vi "CANOpen Edit PDO.vi"(8 "error in (no error)":errorcluster, 11 "Node Ptr":u64 format="%.0x") -> ()   [LabVIEW 2021, in "CANOpen Addon System Explorer.lvlib"]
uses:
  CANOpen Addon System Explorer.lvlib
  SubVIs/CANOpen_PDO Type.ctl
  Shared/CANOpen Addon GUID Lookup Global.vi
  <vilib>/NI VeriStand/Custom Device API/Get Item Property (Variant).vi
  <vilib>/NI VeriStand/Custom Device API/Custom Device API.lvlib
  Shared/CANOpen Addon Shared.lvlib
  <vilib>/NI VeriStand/Custom Device Tools/Custom Device Utility Library/Custom Device Utility Library.lvlib
panel:
  out "error out":errorcluster
  in  "Tag":string
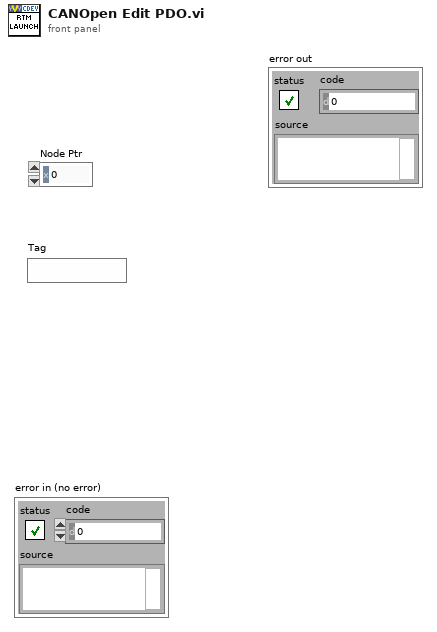
[diagram p1: front panel]
types:
  T1 = typedef "Custom Device API.lvlib/Custom Device Item Info.ctl" = cluster{"Name":string, "Is Channel":bool, "GUID":string, "Is Waveform":bool}
  T2 = typedef "Custom Device API.lvlib/Custom Device Item Ref.ctl" = u64
  T3 = typedef "CANOpen Addon System Explorer.lvlib/CANOpen_PDO Type.ctl" = enum16{"RPDO", "TPDO"}
  T4 = typedef "CANOpen Addon Shared.lvlib/CANOpen_PDO Parameter Settings.ctl" = cluster{"Parameter Name":string, "Scale Factor":dbl, "Scale Offset":dbl, "Byte Offset":u8, "Bit Offset":u8, "Data Type":T5, "Byte Order":T6}
  T5 = typedef "CANOpen Addon Shared.lvlib/CANOpen_PDO Data Type.ctl" = enum16{"U8", "U16", "U32", "I8", "I16", "I32", "Single", "Double", "Boolean"}
  T6 = typedef "CANOpen Addon System Explorer.lvlib/CANopen Byte Order.ctl" = enum16{"big-endian network order", "little-endian"}
  T7 = typedef "CANOpen Addon Shared.lvlib/CANOpen_PDO Settings.ctl" = cluster{"Parameters":T4[], "PDO Channel":u8, "Start Index":u32, "Length":u32}
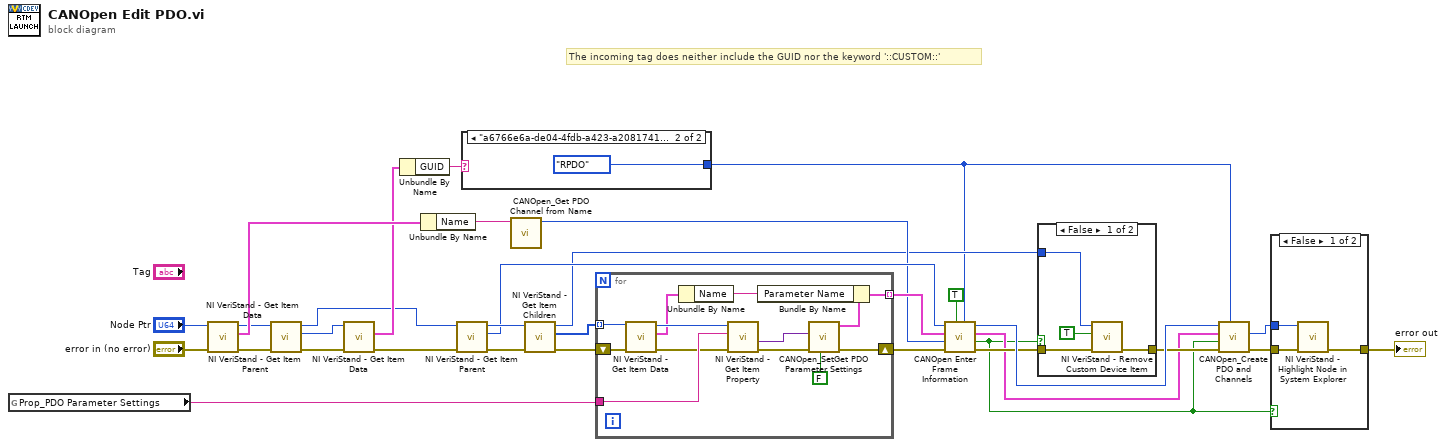
[diagram p0: block diagram]
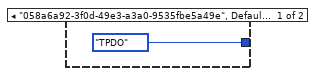
[diagram p2: hidden frame]
diagram:
  # "The incoming tag does neither include the GUID nor the keyword '::CUSTOM::'"
  n1 = global read "CANOpen Addon GUID Lookup Global.vi" "Prop_PDO Parameter Settings"() -> (w30:string)
  n2 = call <vilib>:"NI VeriStand - Get Item Data.vi"("error in (no error)"="error in (no error)", "Item Ref in"="Node Ptr") -> ("error out"=w9:errorcluster, "Item Info"=w26:T1, "Item Ref out"=w8:T2)  [unwired: 7 out]
  n3 = call <vilib>:"NI VeriStand - Get Item Parent.vi"("error in (no error)"=w9, "Item Ref in"=w8) -> ("error out"=w7:errorcluster, "Parent Ref"=w6:T2, "Item Ref out"=w3:T2)  [unwired: 6 in, 1 out]
  n4 = call <vilib>:"NI VeriStand - Get Item Data.vi"("error in (no error)"=w7, "Item Ref in"=w6) -> ("error out"=w2:errorcluster, "Item Info"=w5:T1)  [unwired: 8 out]
  n5 = Unbundle By Name(w5) -> ("GUID"=w4:string)
  n6 = Unbundle By Name(w26) -> ("Name"=w23:string)
  n7 = call <vilib>:"NI VeriStand - Get Item Parent.vi"("error in (no error)"=w2, "Item Ref in"=w3) -> ("error out"=w29:errorcluster, "Parent Ref"=w27:T2, "Item Ref out"=w28:T2)  [unwired: 6 in, 1 out]
  n8 = case shown="\"a6766e6a-de04-4fdb-a423-a2081741c0e8\"" w4 {
    tunnel: [CANOpen_PDO_Type."TPDO" ("Type") CANOpen_PDO_Type."RPDO" ("Type")] -> w1
    frame "058a6a92-3f0d-49e3-a3a0-9535fbe5a49e", Default {
    }
    frame "a6766e6a-de04-4fdb-a423-a2081741c0e8" {
    }
  }
  n9 = call "CANOpen_Get PDO Channel from Name.vi"("PDO Channel Name"=w23) -> ("PDO Channel"=w21:i32)  [unwired: 10 in]
  n10 = call <vilib>:"NI VeriStand - Get Item Children.vi"("error in (no error)"=w29, "Item Ref in"=w28) -> ("error out"=w32:errorcluster, "Child Refs"=w31:T2[], "Item Ref out"=w18:T2)  [unwired: 6 in, 1 out]
  n11 = for {
    shift-right: [w43] -> w19
    shift-left: w32 -> [w42]
    tunnel: w31 -> [w40] mode=indexing
    tunnel: w30 -> [w44]
    tunnel: [w35] -> w22 mode=indexing
    n12 = call <vilib>:"NI VeriStand - Get Item Data.vi"("error in (no error)"=w42, "Item Ref in"=w40) -> ("error out"=w41:errorcluster, "Item Info"=w38:T1, "Item Ref out"=w39:T2)  [unwired: 7 out]
    n13 = Unbundle By Name(w38) -> ("Name"=w37:string)
    n14 = call-poly <vilib>:"NI VeriStand - Get Item Property.vi"("error in (no error)"=w41, "Property Name"=w44, "Item Ref in"=w39) -> ("error out"=w45:errorcluster, "Value"=w46:variant)  [unwired: 5 in, 2 out]
    n15 = call "CANOpen_SetGet PDO Parameter Settings.vi"("Set Parameters"=FALSE, "error in (no error)"=w45, "Parameters"=w46) -> ("error out"=w43:errorcluster, "PDO Parameter Settings out"=w36:T4)  [unwired: 6 in, 1 out]
    n16 = Bundle By Name(cluster=w36, "Parameter Name"=w37) -> (w35:T4)
  }
  n17 = call "CANOpen Enter Frame Information.vi"("Type"=w1, "Edit?"=TRUE, "error in (no error)"=w19, "PDO Channel"=w21, "Parameters"=w22, "Node Ptr"=w27) -> ("error out"=w17:errorcluster, "Cancelled?"=w13:bool, "PDO Settings"=w15:T7, "Item Ref out"=w20:T2)  [unwired: 2 in]
  n18 = case shown="False" w13 {
    tunnel: w18 -> [w50 _]
    tunnel: w17 -> [w49 w52]
    tunnel: [w48 w52] -> w16
    frame False {
      n19 = call <vilib>:"NI VeriStand - Remove Custom Device Item.vi"("error in (no error)"=w49, "Force Delete (F)"=TRUE, "Item Ref in"=w50) -> ("error out"=w48:errorcluster)  [unwired: 7 in, 1 out]
    }
    frame True {
    }
  }
  n20 = call "CANOpen_Create PDO and Channels.vi"("Type"=w1, "error in (no error)"=w16, "Cancelled?"=w13, "PDO Settings"=w15, "Item Ref out"=w20) -> ("error out"=w11:errorcluster, "New PDO"=w10:T2)  [unwired: 5 in]
  n21 = case shown="False" w13 {
    tunnel: [w54 w56] -> w12
    tunnel: w11 -> [w55 w56]
    tunnel: w10 -> [w53 _]
    frame False {
      n22 = call <vilib>:"NI VeriStand - Highlight Node in System Explorer.vi"("error in (no error)"=w55, "Item Ref in"=w53) -> ("error out"=w54:errorcluster)  [unwired: 8 in, 1 out]
    }
    frame True {
    }
  }
  "error out" <- w12
